vi "Upload Serial Number.vi"(5 "timeout ms (-1)":i32=-1, 6 "Station":T1(ring), 7 "Socket":i32, 8 "error in (no error)":errorcluster, 11 "SerialNumber":string) -> (0 "error out":errorcluster)   [LabVIEW 2019, in "Unit Test Engine Tools.lvlib"]
uses:
  Unit Test Engine Tools.lvlib
  LVUT Global 1.vi
  <resource>/objmgr/ni.dex.rc
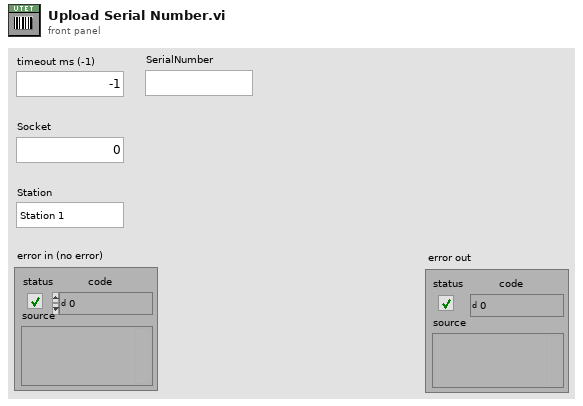
[diagram p1: front panel]
types:
  T1 = enum16{"Station 1", "Station 2", "Station 3", "Station 4"}
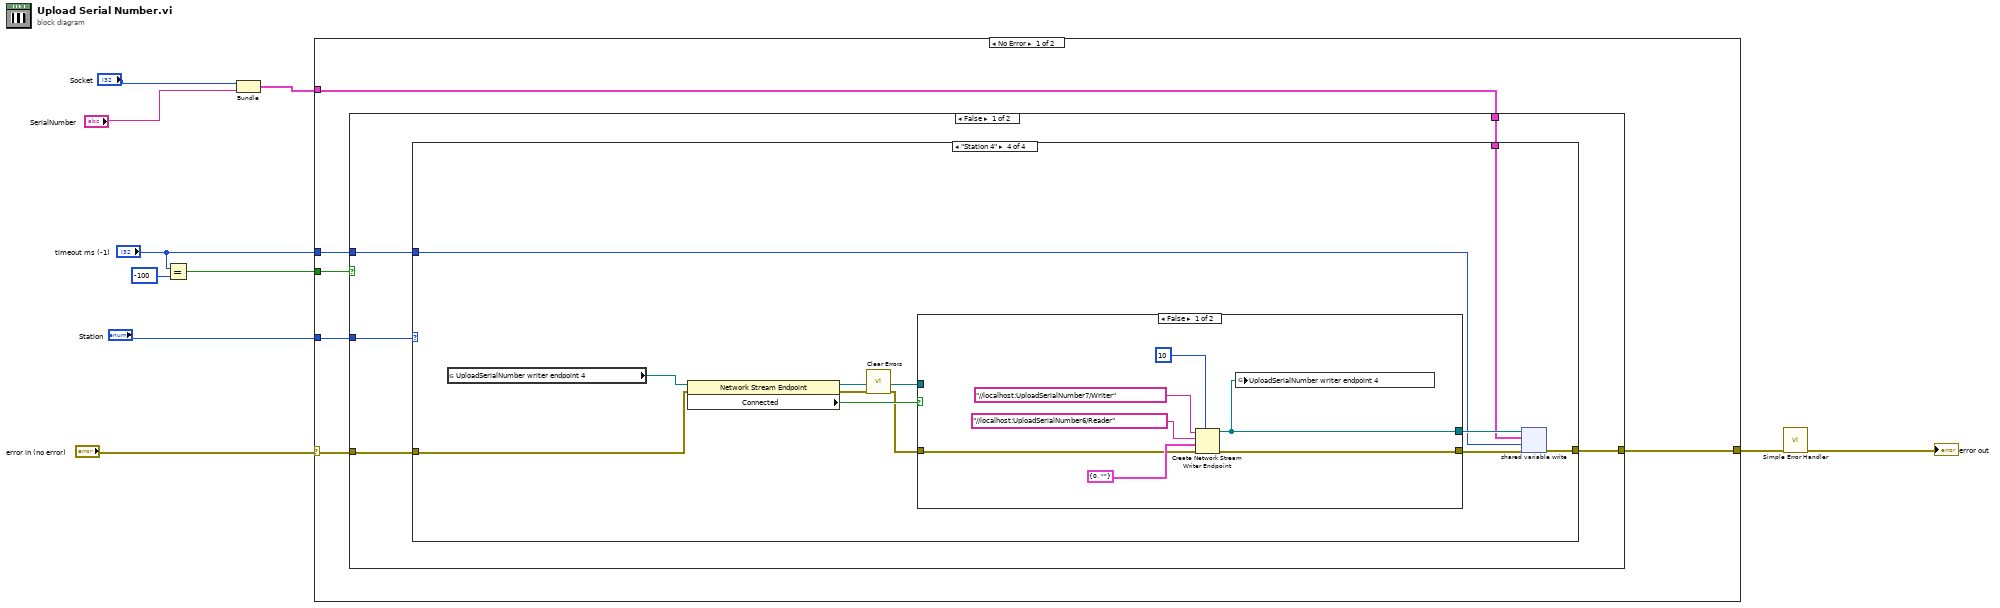
[diagram p0: block diagram]
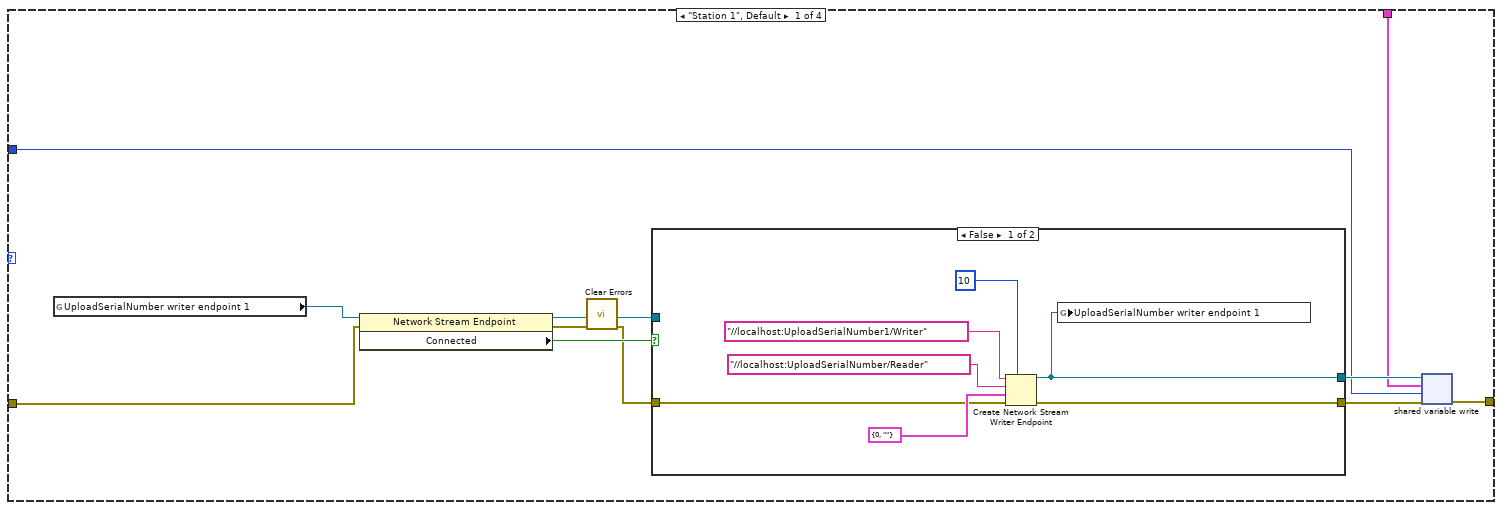
[diagram p2: hidden frame]
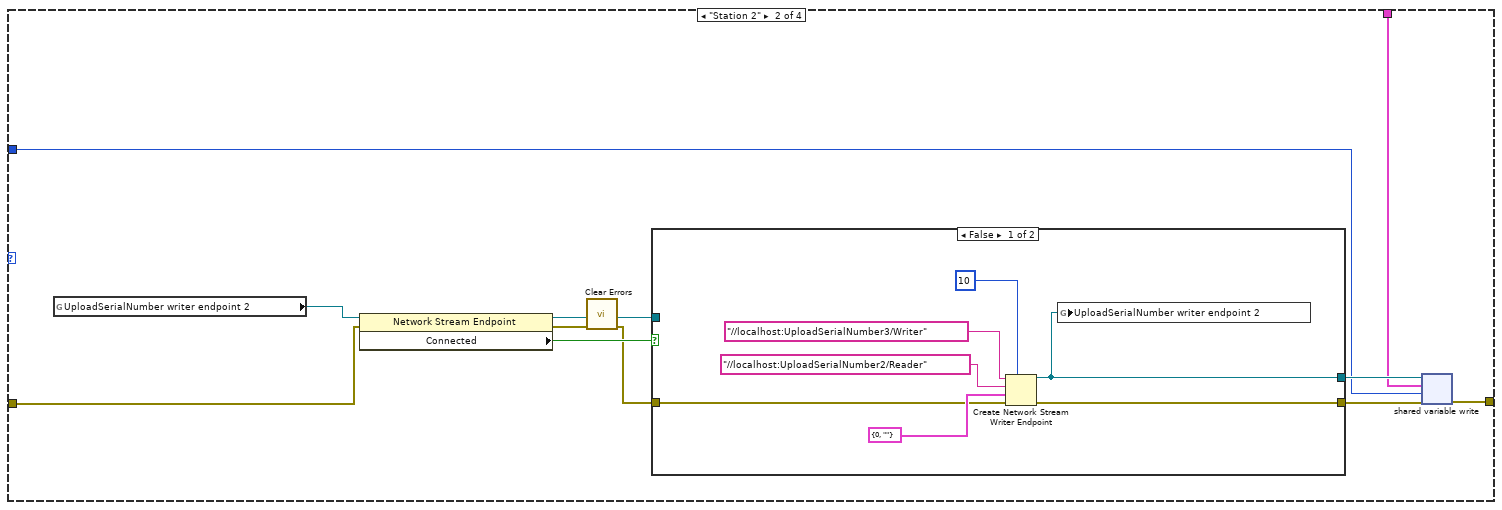
[diagram p4: hidden frame]
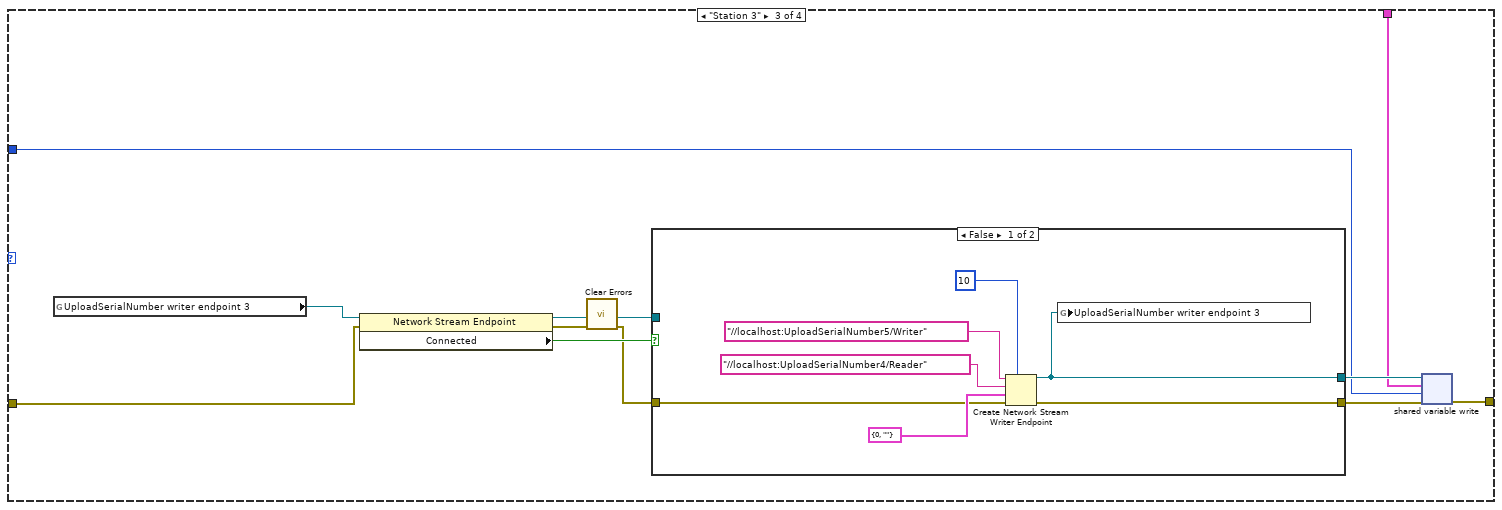
[diagram p6: hidden frame]
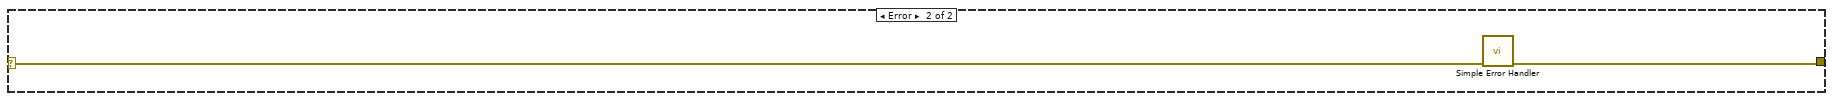
[diagram p10: hidden frame]
diagram:
  n1 = Equal?(x="timeout ms (-1)", y=-100) -> (x = y?=w1:bool)
  n2 = Bundle("Socket"="Socket", "SerialNumber"="SerialNumber") -> (w10:cluster{"Socket":i32, "SerialNumber":string})  [unwired: 1 in]
  n3 = case shown="No Error" "error in (no error)" {
    selector: "error in (no error)" -> [w13 w104]
    tunnel: "timeout ms (-1)" -> [w16 _]
    tunnel: w10 -> [w15 _]
    tunnel: [w14 w103] -> w9
    tunnel: "Station" -> [w12 _]
    tunnel: w1 -> [w11 _]
    frame No Error {
      n4 = case shown="False" w11 {
        tunnel: w16 -> [w21 _]
        tunnel: w15 -> [w20 _]
        tunnel: [w19 w102] -> w14
        tunnel: w13 -> [w18 w102]
        tunnel: w12 -> [w17 _]
        frame False {
          n5 = case shown="\"Station 4\"" w17 {
            tunnel: w21 -> [w30 w50 w70 w90]
            tunnel: w20 -> [w29 w49 w69 w89]
            tunnel: [w24 w44 w64 w84] -> w19
            tunnel: w18 -> [w23 w43 w63 w83]
            frame "Station 1", Default {
              n6 = global read "LVUT Global 1.vi" "UploadSerialNumber writer endpoint 1"() -> (w28:refnum<k21>)
              n7 = property class="Network Stream Endpoint"(reference=w28, error in=w23) -> (reference out=w25:refnum<k21>, error out=w27:errorcluster, "Connected"=w26:bool)
              n8 = call <vilib>:"Clear Errors.vi"("error in (no error)"=w27) -> ("error out"=w22:errorcluster)  [unwired: 5 in, 1 out]
              n9 = case shown="False" w26 {
                tunnel: [w33 w41] -> w32
                tunnel: [w36 w40] -> w31
                tunnel: w22 -> [w34 w40]
                tunnel: w25 -> [_ w41]
                frame False {
                  n10 = Create Network Stream Writer Endpoint(7:10 ("writer buffer size"), 8:w34, 9:cluster{"Socket":i32, "SerialNumber":string} {"Socket"=0, "SerialNumber"=""}, 10:"//localhost:UploadSerialNumber/Reader" ("reader name"), 11:"//localhost:UploadSerialNumber1/Writer" ("reader name")) -> (0:w36:errorcluster, 3:w33:refnum<k21>)  [unwired: 2 in]
                  n11 = global write "LVUT Global 1.vi" "UploadSerialNumber writer endpoint 1"(w33) -> ()
                }
                frame True {
                }
              }
              n12 = shared-variable-write(w32, w31, w29, w30) -> (w24:errorcluster)  [unwired: 2 out]
            }
            frame "Station 2" {
              n13 = global read "LVUT Global 1.vi" "UploadSerialNumber writer endpoint 2"() -> (w48:refnum<k21>)
              n14 = property class="Network Stream Endpoint"(reference=w48, error in=w43) -> (reference out=w45:refnum<k21>, error out=w47:errorcluster, "Connected"=w46:bool)
              n15 = call <vilib>:"Clear Errors.vi"("error in (no error)"=w47) -> ("error out"=w42:errorcluster)  [unwired: 5 in, 1 out]
              n16 = case shown="False" w46 {
                tunnel: [w53 w61] -> w52
                tunnel: [w56 w60] -> w51
                tunnel: w42 -> [w54 w60]
                tunnel: w45 -> [_ w61]
                frame False {
                  n17 = Create Network Stream Writer Endpoint(7:10 ("writer buffer size"), 8:w54, 9:cluster{"Socket":i32, "SerialNumber":string} {"Socket"=0, "SerialNumber"=""}, 10:"//localhost:UploadSerialNumber2/Reader" ("reader name"), 11:"//localhost:UploadSerialNumber3/Writer" ("reader name")) -> (0:w56:errorcluster, 3:w53:refnum<k21>)  [unwired: 2 in]
                  n18 = global write "LVUT Global 1.vi" "UploadSerialNumber writer endpoint 2"(w53) -> ()
                }
                frame True {
                }
              }
              n19 = shared-variable-write(w52, w51, w49, w50) -> (w44:errorcluster)  [unwired: 2 out]
            }
            frame "Station 3" {
              n20 = global read "LVUT Global 1.vi" "UploadSerialNumber writer endpoint 3"() -> (w68:refnum<k21>)
              n21 = property class="Network Stream Endpoint"(reference=w68, error in=w63) -> (reference out=w65:refnum<k21>, error out=w67:errorcluster, "Connected"=w66:bool)
              n22 = call <vilib>:"Clear Errors.vi"("error in (no error)"=w67) -> ("error out"=w62:errorcluster)  [unwired: 5 in, 1 out]
              n23 = case shown="False" w66 {
                tunnel: [w73 w81] -> w72
                tunnel: [w76 w80] -> w71
                tunnel: w62 -> [w74 w80]
                tunnel: w65 -> [_ w81]
                frame False {
                  n24 = Create Network Stream Writer Endpoint(7:10 ("writer buffer size"), 8:w74, 9:cluster{"Socket":i32, "SerialNumber":string} {"Socket"=0, "SerialNumber"=""}, 10:"//localhost:UploadSerialNumber4/Reader" ("reader name"), 11:"//localhost:UploadSerialNumber5/Writer" ("reader name")) -> (0:w76:errorcluster, 3:w73:refnum<k21>)  [unwired: 2 in]
                  n25 = global write "LVUT Global 1.vi" "UploadSerialNumber writer endpoint 3"(w73) -> ()
                }
                frame True {
                }
              }
              n26 = shared-variable-write(w72, w71, w69, w70) -> (w64:errorcluster)  [unwired: 2 out]
            }
            frame "Station 4" {
              n27 = global read "LVUT Global 1.vi" "UploadSerialNumber writer endpoint 4"() -> (w88:refnum<k21>)
              n28 = property class="Network Stream Endpoint"(reference=w88, error in=w83) -> (reference out=w85:refnum<k21>, error out=w87:errorcluster, "Connected"=w86:bool)
              n29 = call <vilib>:"Clear Errors.vi"("error in (no error)"=w87) -> ("error out"=w82:errorcluster)  [unwired: 5 in, 1 out]
              n30 = case shown="False" w86 {
                tunnel: [w93 w101] -> w92
                tunnel: [w96 w100] -> w91
                tunnel: w82 -> [w94 w100]
                tunnel: w85 -> [_ w101]
                frame False {
                  n31 = Create Network Stream Writer Endpoint(7:10 ("writer buffer size"), 8:w94, 9:cluster{"Socket":i32, "SerialNumber":string} {"Socket"=0, "SerialNumber"=""}, 10:"//localhost:UploadSerialNumber6/Reader" ("reader name"), 11:"//localhost:UploadSerialNumber7/Writer" ("reader name")) -> (0:w96:errorcluster, 3:w93:refnum<k21>)  [unwired: 2 in]
                  n32 = global write "LVUT Global 1.vi" "UploadSerialNumber writer endpoint 4"(w93) -> ()
                }
                frame True {
                }
              }
              n33 = shared-variable-write(w92, w91, w89, w90) -> (w84:errorcluster)  [unwired: 2 out]
            }
          }
        }
        frame True {
        }
      }
    }
    frame Error {
      n34 = call <vilib>:"Simple Error Handler.vi"("error in (no error)"=w104) -> ("error out"=w103:errorcluster)  [unwired: 4 in, 4 out]
    }
  }
  n35 = call <vilib>:"Simple Error Handler.vi"("error in (no error)"=w9) -> ("error out"=→"error out":errorcluster)  [unwired: 4 in, 4 out]
